vi "Write Start Index.vi"(8 "error in (no error)":errorcluster, 10 "Start Index":i32, 11 "Set Ratios Msg in":refnum<class "Set Ratios Msg.lvclass">) -> (0 "error out":errorcluster, 3 "Set Ratios Msg out":refnum<class "Set Ratios Msg.lvclass">)   [LabVIEW 2021, in "BNT_ULx.lvlib" / "Set Ratios Msg.lvclass"]
uses:
  Set Ratios Msg.lvclass
  Set Ratios Msg.lvclass/Set Ratios Msg.ctl
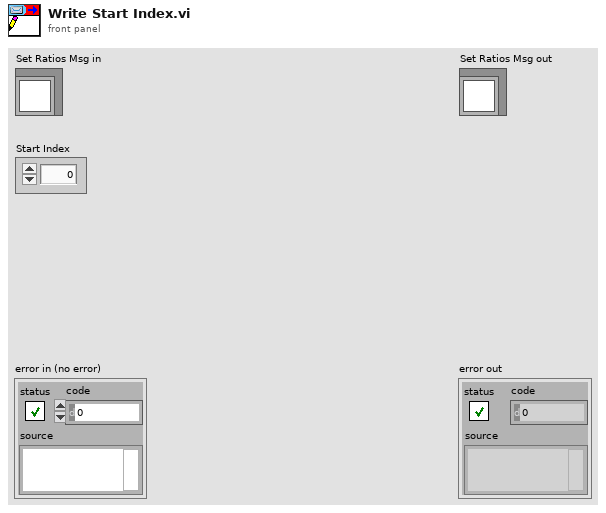
[diagram p1: front panel]
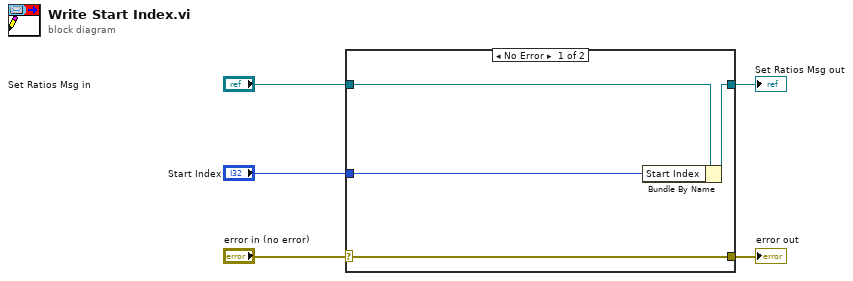
[diagram p0: block diagram]
diagram:
  n1 = case shown="No Error" "error in (no error)" {
    selector: "error in (no error)" -> [w9 w10]
    tunnel: [w9 w10] -> w4
    tunnel: [w7 w11] -> w2
    tunnel: "Set Ratios Msg in" -> [w8 w11]
    tunnel: "Start Index" -> [w6 _]
    frame No Error {
      n2 = Bundle By Name(cluster=w8, "Start Index"=w6) -> (w7:refnum<class "Set Ratios Msg.lvclass">)
    }
    frame Error {
    }
  }
  "error out" <- w4
  "Set Ratios Msg out" <- w2
